vi "Auton Drive Ramper2.vi"(9 "Target Setpoint":dbl, 11 "Rate":dbl) -> (1 "Ramping":bool, 3 "Current Setpoint":dbl)   [LabVIEW 2011]
panel:
  out "crement":dbl
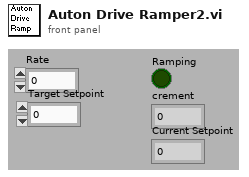
[diagram p1: front panel]
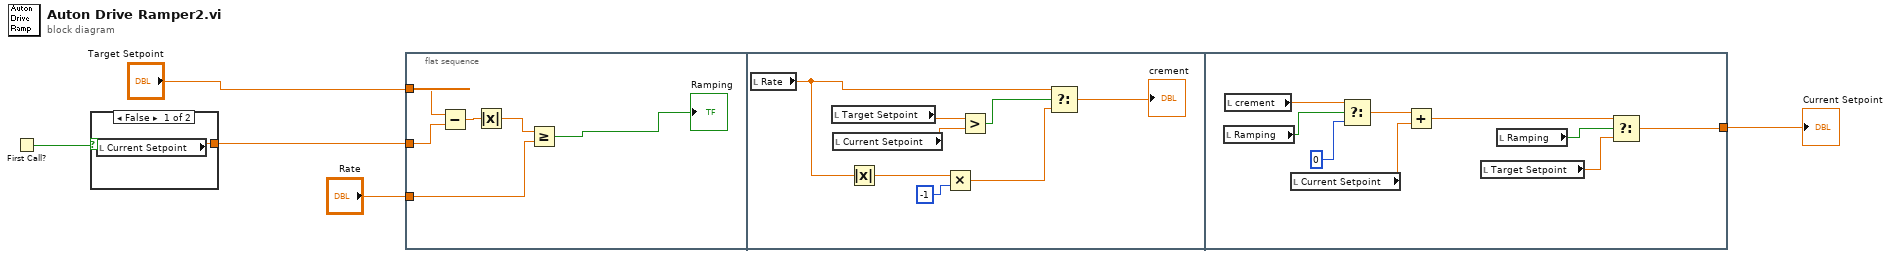
[diagram p0: block diagram]
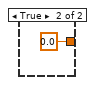
[diagram p2: hidden frame]
diagram:
  n1 = First Call?() -> (First Call?: T/F=w1:bool)
  n2 = case shown="False" w1 {
    tunnel: [w6 0.0 ("Current Setpoint")] -> w2
    frame False {
      n3 = local read "Current Setpoint"() -> (w6:dbl)
    }
    frame True {
    }
  }
  n4 = flat-sequence {
    tunnel: "Target Setpoint" -> [w9]
    tunnel: w2 -> [w11]
    tunnel: "Rate" -> [w10]
    tunnel: [w24] -> w4
    frame #0 {
      n5 = Subtract(x=w9, y=w11) -> (x-y=w12:dbl)
      n6 = Absolute Value(x=w12) -> (abs(x)=w13:dbl)
      n7 = Greater Or Equal?(x=w13, y=w10) -> (x >= y?=→"Ramping":bool)
    }
    frame #1 {
      n8 = local read "Rate"() -> (w18:dbl)
      n9 = local read "Target Setpoint"() -> (w21:dbl)
      n10 = local read "Current Setpoint"() -> (w20:dbl)
      n11 = Absolute Value(x=w18) -> (abs(x)=w17:dbl)
      n12 = Multiply(x=w17, y=-1) -> (x*y=w15:dbl)
      n13 = Greater?(x=w21, y=w20) -> (0:w19:bool)
      n14 = Select(t=w18, s=w19, f=w15) -> (s? t:f=→"crement":dbl)
    }
    frame #2 {
      n15 = local read "Ramping"() -> (w29:bool)
      n16 = local read "crement"() -> (w30:dbl)
      n17 = local read "Current Setpoint"() -> (w22:dbl)
      n18 = Select(t=w30, s=w29, f=0) -> (s? t:f=w27:dbl)
      n19 = Add(x=w27, y=w22) -> (x+y=w26:dbl)
      n20 = local read "Target Setpoint"() -> (w25:dbl)
      n21 = local read "Ramping"() -> (w23:bool)
      n22 = Select(t=w26, s=w23, f=w25) -> (s? t:f=w24:dbl)
    }
  }
  "Current Setpoint" <- w4
